vi "Create QControl Directory.vi"(8 "Error In":errorcluster, 11 "Path":path) -> (0 "Error Out":errorcluster, 3 "Duplicate Path":path)   [LabVIEW 2020, in "QControl Creation.lvclass"]
doc: "<b> </b> <b> </b>\n©2016 Q Software Innovations, LLC (QSI)\nwritten by Quentin Alldredge\nproduced in LabVIEW 2015\n\nsupport@qsoftwareinnovations.com\nwww.qsoftwareinnovations.com\n\nAll rights reserved.\n\nRedistribution and use in source and binary forms, with or without modification, are permitted provided that the following conditions are met:\n\n * Redistributions of source code must retain the above copyright notice, this list of conditions and the following disclaimer.\n * Redistributions in binary form must reproduce the above copyright notice, this list of conditions and the following disclaimer in the documentation and/or other materials provided with the distribution.\n * Neither the name of Q Software Innovations, LLC. nor the names of its contributors may be used to endorse or promote products derived from this software without specific prior written permission.\n\nTHIS SOFTWARE IS PROVIDED BY THE COPYRIGHT HOLDERS AND CONTRIBUTORS \"AS IS\" AND ANY EXPRESS OR IMPLIED WARRANTIES, INCLUDING, BUT NOT LIMITED TO, THE IMPLIED WARRANTIES OF MERCHANTABILITY AND FITNESS FOR A PARTICULAR PURPOSE ARE DISCLAIMED. IN NO EVENT SHALL THE COPYRIGHT OWNER OR CONTRIBUTORS BE LIABLE FOR ANY DIRECT, INDIRECT, INCIDENTAL, SPECIAL, EXEMPLARY, OR CONSEQUENTIAL DAMAGES (INCLUDING, BUT NOT LIMITED TO, PROCUREMENT OF SUBSTITUTE GOODS OR SERVICES; LOSS OF USE, DATA, OR PROFITS; OR BUSINESS INTERRUPTION) HOWEVER CAUSED AND ON ANY THEORY OF LIABILITY, WHETHER IN CONTRACT, STRICT LIABILITY, OR TORT (INCLUDING NEGLIGENCE OR OTHERWISE) ARISING IN ANY WAY OUT OF THE USE OF THIS SOFTWARE, EVEN IF ADVISED OF THE POSSIBILITY OF SUCH DAMAGE."
uses:
  QControl Creation.lvclass
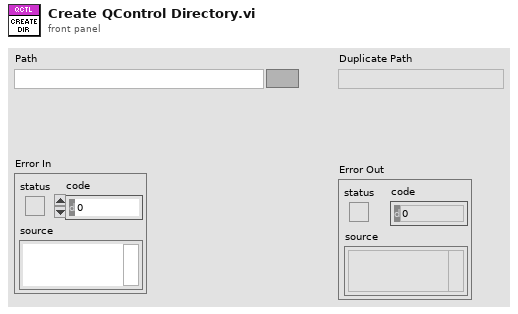
[diagram p1: front panel]
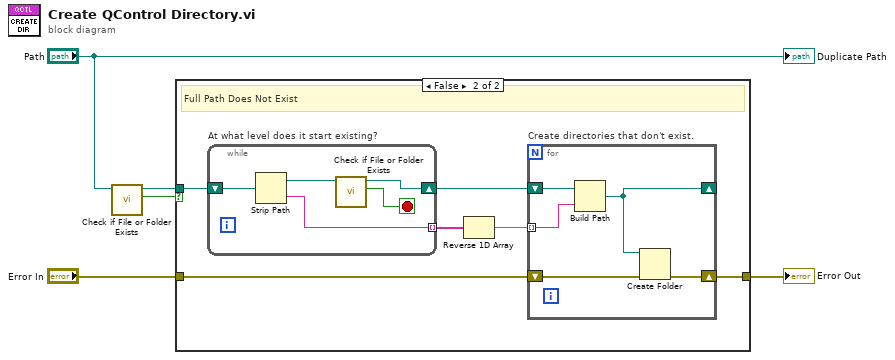
[diagram p0: block diagram]
diagram:
  n1 = call <vilib>:"Check if File or Folder Exists.vi"("path"="Path") -> ("file or folder exists?"=w1:bool, "dup path"=w2:path)  [unwired: 8 in, 1 out]
  n2 = case shown="False" w1 {
    tunnel: "Error In" -> [w6 w10]
    tunnel: [w6 w7] -> w5
    tunnel: w2 -> [_ w9]
    frame True {
      # "Exists.  Do Nothing."
    }
    frame False {
      # "Full Path Does Not Exist"
      n3 = while "At what level does it start existing?" {
        shift-right: [w14] -> w11
        shift-left: w9 -> [w17]
        tunnel: [w15] -> w12 mode=indexing
        stop <- w13 stop-if-true
        n4 = Strip Path(path=w17) -> (stripped path=w16:path, name=w15:string)
        n5 = call <vilib>:"Check if File or Folder Exists.vi"("path"=w16) -> ("file or folder exists?"=w13:bool, "dup path"=w14:path)  [unwired: 8 in, 1 out]
      }
      n6 = Reverse 1D Array(array=w12) -> (reversed array=w8:string[])
      n7 = for "Create directories that don't exist." {
        shift-right: [w18] -> _
        shift-left: w11 -> [w22]
        tunnel: w8 -> [w21] mode=indexing
        shift-right: [w19] -> w7
        shift-left: w10 -> [w20]
        n8 = Build Path(base path=w22, name or relative path=w21) -> (appended path=w18:path)
        n9 = Create Folder(path (use dialog)=w18, error in=w20) -> (error out=w19:errorcluster)  [unwired: 1 in, 2 out]
      }
    }
  }
  "Error Out" <- w5
  "Duplicate Path" <- "Path"
